vi "Analog Tach Process.vi"(4 "slope (Rise)":enum16{"Rise", "Fall"}(ring), 5 "reset? (True)":bool=TRUE, 6 "pulse width (2)":i32=2, 7 "missing pulses? (no:F)":bool, 8 "avg on n pulses (1:no average)":i32=1, 9 "pulse/revolution (1)":i32=1, 10 "threshold (auto)":dbl=inf format="%.2f", 11 "analog tach signal":waveform(dbl)={"t0"=timestamp(0 s since 1904-01-01), "dt"=0.0, "Y"=[]}) -> (0 "error out":errorcluster, 1 "pulse positions [s]":dbl[](array[numeric]) format="%.2f", 3 "speed profile":T1 {"speed [RPM]" format="%.2f"; "time [s]" format="%.2f"})   [LabVIEW 2017, in "SoundVib_TachProcess.lvlib"]
doc: "Processes well-conditioned analog tachometer signals, such as those in which there is no trend involved."
uses:
  <vilib>/addons/Sound and Vibration/Order Analysis/Tach Process/SoundVib_TachProcess.lvlib
  <vilib>/addons/Sound and Vibration/Order Analysis/Tach Process/SubVIs/speed profile.ctl
panel:
  # "Analog Tach Process"
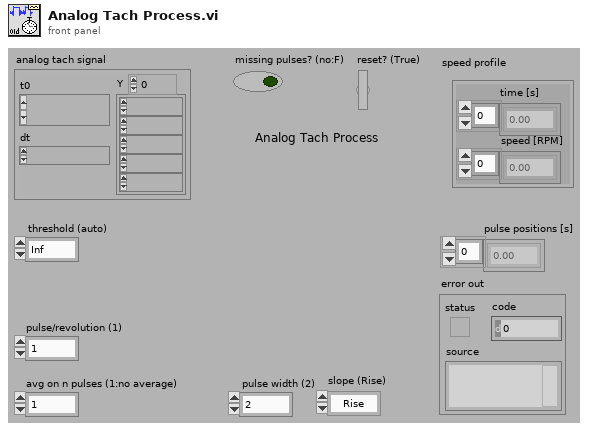
[diagram p1: front panel]
types:
  T1 = typedef "SoundVib_TachProcess.lvlib/speed profile.ctl" = cluster{"time [s]":dbl[], "speed [RPM]":dbl[]}
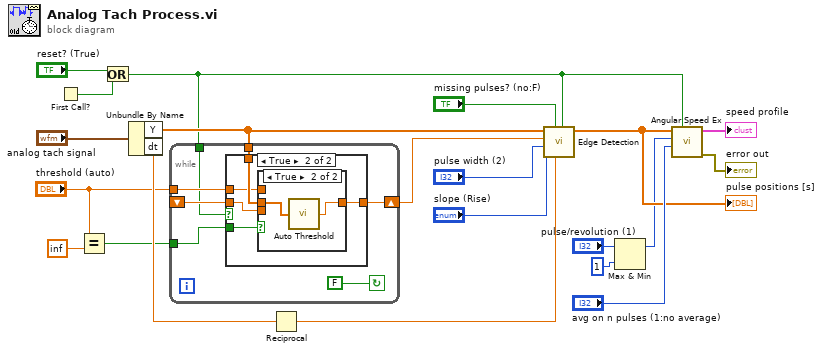
[diagram p0: block diagram]
diagram:
  n1 = First Call?() -> (First Call?: T/F=w10:bool)
  n2 = Equal?(x="threshold (auto)", y=inf) -> (x = y?=w6:bool)
  n3 = Or(x="reset? (True)", y=w10) -> (x .or. y?=w1:bool)
  n4 = Unbundle By Name("analog tach signal") -> ("Y"=w12:dbl[], "dt"=w14:dbl)
  n5 = while {
    tunnel: w12 -> [w28]
    shift-right: [w27] -> w11
    shift-left: _ -> [w26]
    tunnel: w1 -> [w23]
    tunnel: w6 -> [w22]
    tunnel: "threshold (auto)" -> [w24]
    stop <- FALSE continue-if-true
    n6 = case shown="True" w23 {
      tunnel: w28 -> [_ w34]
      tunnel: [w29 w33] -> w27
      tunnel: w26 -> [w29 w32]
      tunnel: w24 -> [_ w31]
      tunnel: w22 -> [_ w30]
      frame False {
      }
      frame True {
        n7 = case shown="True" w30 {
          tunnel: w34 -> [_ w37]
          tunnel: [w35 w36] -> w33
          tunnel: w32 -> [_ _]
          tunnel: w31 -> [w35 _]
          frame False {
          }
          frame True {
            n8 = call <vilib>:"Auto Threshold.vi"("x[n]"=w37) -> ("threshold"=w36:dbl)
          }
        }
      }
    }
  }
  n9 = Reciprocal(x=w14) -> (1/x=w13:dbl)
  n10 = call <vilib>:"Edge Detection.vi"("reset? (True)"=w1, "sampling frequency [Hz]"=w13, "missing pulses? (no:F)"="missing pulses? (no:F)", "slope (Rise)"="slope (Rise)", "pulse width (2)"="pulse width (2)", "threshold (0.0)"=w11, "x[n]"=w12) -> ("pulse positions [s]"=w15:dbl[])  [unwired: 3 in, 1 out]
  "pulse positions [s]" <- w15
  n11 = Max & Min(x="pulse/revolution (1)", y=1) -> (max(x,y)=w3:i32)  [unwired: 1 out]
  n12 = call <vilib>:"Angular Speed Ex.vi"("reset? (True)"=w1, "avg on n pulses (1:no average)"="avg on n pulses (1:no average)", "pulse/revolution (1)"=w3, "pulse positions [s]"=w15) -> ("error out"=→"error out":errorcluster, "speed profile"=→"speed profile":T1)  [unwired: 6 in]
